vi "运维调试.vi"   [LabVIEW 2016]
uses:
  <vilib>/Utility/config.llb/NI_LVConfig.lvlib
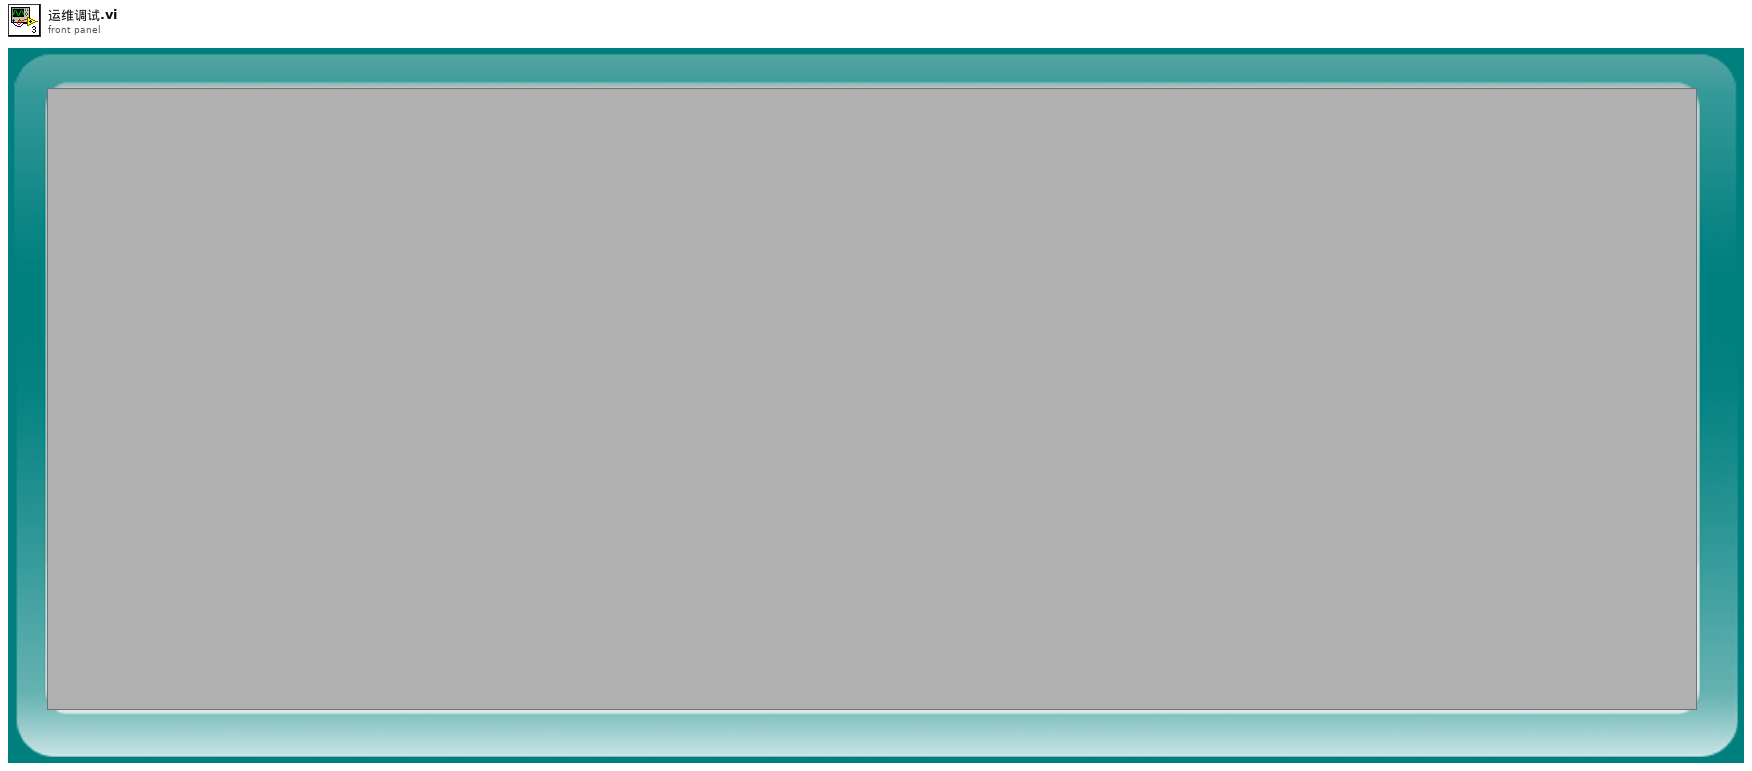
[diagram p1: front panel]
types:
  T1 = typedef "NI_LVConfig.lvlib/Config Data RefNum.ctl" = refnum<k1>
  T2 = enum32{"Bad", "Idle", "Run top level", "Running"}
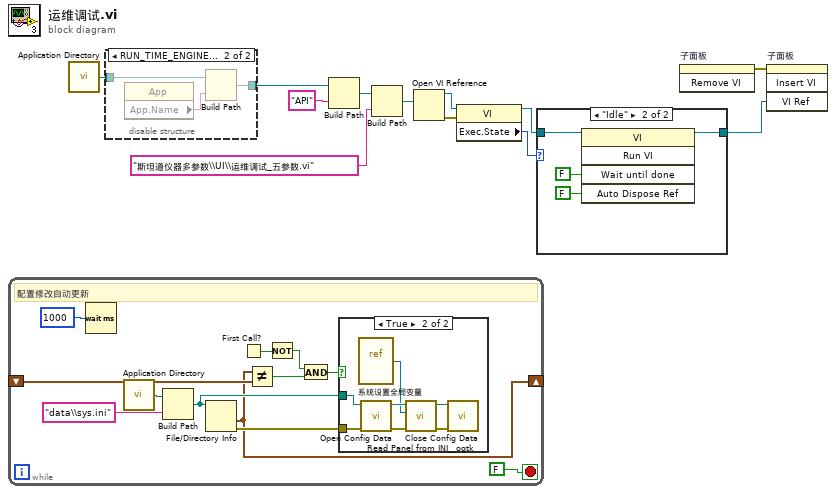
[diagram p0: block diagram]
diagram:
  n1 = while {
    shift-right: [w16] -> _
    shift-left: _ -> [w19]
    stop <- FALSE stop-if-true
    # "配置修改自动更新"
    n2 = Wait (ms)(milliseconds to wait=u32 1000 ("等待时间（毫秒）")) -> ()  [unwired: 1 out]
    n3 = call <vilib>:"Application Directory.vi"() -> ("Application Directory"=w22:path)
    n4 = Build Path(base path=w22, name or relative path="data\\sys.ini" ("名称或相对路径")) -> (appended path=w20:path)
    n5 = File/Directory Info(path=w20) -> (last mod=w16:timestamp, error out=w17:errorcluster)  [unwired: 1 in, 5 out]
    n6 = First Call?() -> (First Call?: T/F=w14:bool)
    n7 = Not Equal?(x=w16, y=w19) -> (x != y?=w18:bool)
    n8 = Not(x=w14) -> (.not. x?=w13:bool)
    n9 = And(x=w13, y=w18) -> (x .and. y?=w15:bool)
    n10 = case shown="True" w15 {
      tunnel: w20 -> [_ w26]
      tunnel: w17 -> [_ w25]
      frame False {
      }
      frame True {
        n11 = vi-ref "系统设置全局变量.vi"() -> (w29:refnum<vi>)
        n12 = call <vilib>:"Open Config Data.vi"("error in (no error)"=w25, "configuration file path"=w26) -> ("error out"=w31:errorcluster, "refnum"=w30:T1)  [unwired: 7 in, 1 out]
        n13 = call <userlib>:"Read Panel from INI__ogtk.vi"("error in (no error)"=w31, "VI ref"=w29, "refnum"=w30) -> ("error out"=w28:errorcluster, "refnum out"=w27:T1)  [unwired: 7 in]
        n14 = call <vilib>:"Close Config Data.vi"("error in (no error)"=w28, "refnum"=w27) -> ()  [unwired: 8 in, 2 out]
      }
    }
  }
  n15 = call <vilib>:"Application Directory.vi"() -> ("Application Directory"=w12:path)
  n16 = disable-structure shown="RUN_TIME_ENGINE==True" {
    disable-tunnel: w12 -> [w32 w35]
    disable-tunnel: [w32 w33] -> w10
    frame condition #0 (active) {
    }
    frame condition #1 {
      n17 = property class="App"() -> ("App.Name"=w34:string)  [unwired: 2 in, 2 out]
      n18 = Build Path(base path=w35, name or relative path=w34) -> (appended path=w33:path)
    }
  }
  n19 = Build Path(base path=w10, name or relative path="API" ("名称或相对路径")) -> (appended path=w7:path)
  n20 = Build Path(base path=w7, name or relative path="斯坦道仪器多参数\\UI\\运维调试_五参数.vi" ("名称或相对路径")) -> (appended path=w2:path)
  n21 = Open VI Reference(vi path=w2) -> (vi reference=w4:refnum<vi>, error out=w5:errorcluster)  [unwired: 5 in]
  n22 = property class="VI"(reference=w4, error in=w5) -> (reference out=w6:refnum<vi>, "Exec.State"=w3:T2)  [unwired: 1 out]
  n23 = case shown="\"Idle\"" w3 {
    tunnel: w6 -> [w36 w38]
    tunnel: [w36 w37] -> w1
    frame "Bad", Default {
    }
    frame "Idle" {
      n24 = invoke class="VI" method="Run VI"(reference=w38, "Wait until done"=FALSE ("结束前等待"), "Auto Dispose Ref"=FALSE ("自动销毁引用")) -> (reference out=w37:refnum<vi>)  [unwired: 2 in, 4 out]
    }
  }
  n25 = invoke on="子面板" class="SubPnl" method="Remove VI"() -> (error out=w8:errorcluster)  [unwired: 3 in, 2 out]
  n26 = invoke on="子面板" class="SubPnl" method="Insert VI"(error in=w8, "VI Ref"=w1) -> ()  [unwired: 2 in, 4 out]
